vi "Image (Mask) SGL Data.vi"(8 "error in (no error)":errorcluster, 10 "Image Mask Refnum":T2, 11 "Src Image Refnum":T2) -> (0 "error out":errorcluster, 1 "% of Image":dbl, 2 "[Pixel Coordinates]":T1[](array[typedef]), 3 "Pixel Values(Float)":sgl[](array[numeric]), 4 "# Mask Pixels":i32, 5 "CPU (s)":dbl)   [LabVIEW 2021]
doc: "Returns the value (SGL) of pixels od the <B>Src Image</B> matching the mask.\n<B>Image Mask</B> needs to be of U8 or U16 type."
uses:
  <vilib>/vision/Image Controls.llb/IMAQ Image.ctl
  Image Point.ctl
  <vilib>/vision/NI_Vision_Development_Module.lvlib
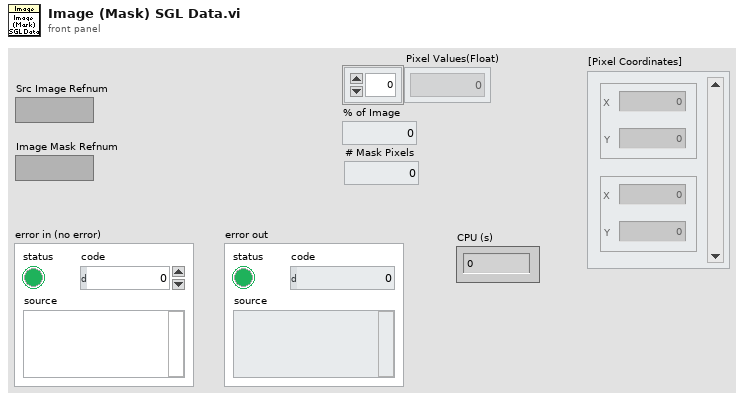
[diagram p1: front panel]
types:
  T1 = typedef "Image Point.ctl" = cluster{"X":i32, "Y":i32}
  T2 = typedef "IMAQ Image.ctl" = refnum<image>
  T3 = typedef "Image Type" = u32
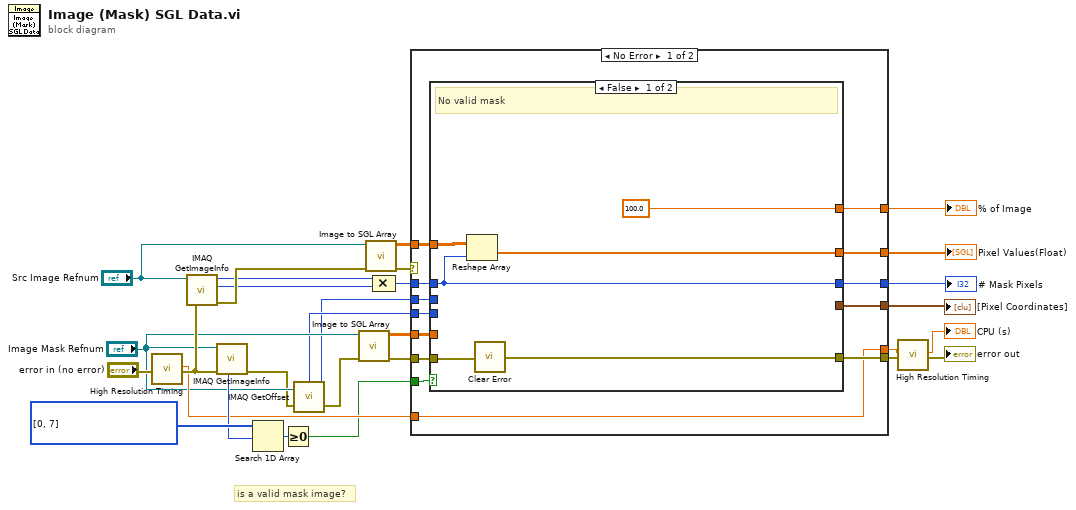
[diagram p0: block diagram]
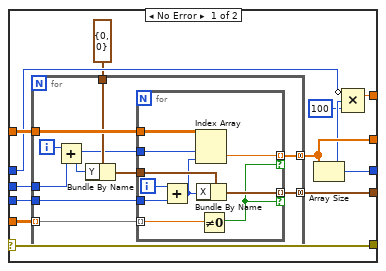
[diagram p3: hidden frame]
diagram:
  w29 = T3[] [0, 7] items=["Grayscale (U8)", "Grayscale (I16)", "Grayscale (SGL)", "Complex (CSG)", "RGB (U32)", "HSL (U32)", "RGB (U64)", "Grayscale (U16)"] ("Array")
  # "is a valid mask image?"
  n1 = call "High Resolution Timing.vi"("Error In"="error in (no error)") -> ("elapsed (relative) seconds"=w13:dbl, "Error Out"=w17:errorcluster)  [unwired: 16 in, 1 out]
  n2 = call "IMAQ GetImageInfo"("error in (no error)"=w17, "Image"="Src Image Refnum") -> ("error out"=w26:errorcluster, "Y Resolution"=w23:i32, "X Resolution"=w24:i32)  [unwired: 2 in, 5 out]
  n3 = call "IMAQ GetImageInfo"("error in (no error)"=w17, "Image"="Image Mask Refnum") -> ("error out"=w9:errorcluster, "Image Type"=w28:T3)  [unwired: 2 in, 6 out]
  n4 = Search 1D Array(1D array=w29, element=w28) -> (index of element=w27:i32)  [unwired: 1 in]
  n5 = Greater Or Equal To 0?(x=w27) -> (x >= 0?=w5:bool)
  n6 = call "IMAQ GetOffset"("Image"="Image Mask Refnum", "error in (no error)"=w9) -> ("Y Offset"=w7:i32, "X Offset"=w8:i32, "error out"=w6:errorcluster)  [unwired: 2 in]
  n7 = call "Image to SGL Array.vi"("error in (no error)"=w6, "Image"="Image Mask Refnum") -> ("error out"=w22:errorcluster, "Image Pixels (Float)"=w19:sgl[][])  [unwired: 8 in]
  n8 = call "Image to SGL Array.vi"("error in (no error)"=w26, "Image"="Src Image Refnum") -> ("error out"=w16:errorcluster, "Image Pixels (Float)"=w21:sgl[][])  [unwired: 8 in]
  n9 = Compound Arithmetic op=MULTIPLY(w24, w23) -> (w20:i32)
  n10 = case shown="No Error" w16 {
    selector: w16 -> [_ w95]
    tunnel: w5 -> [w42 _]
    tunnel: w22 -> [w41 _]
    tunnel: w21 -> [w38 _]
    tunnel: w20 -> [w40 _]
    tunnel: w19 -> [w39 _]
    tunnel: [w35 w95] -> w15
    tunnel: [w34 w94] -> w12
    tunnel: w13 -> [w34 w94]
    tunnel: w8 -> [w36 _]
    tunnel: w7 -> [w37 _]
    tunnel: [w33 _] -> w4
    tunnel: [w32 _] -> w3
    tunnel: [w31 _] -> w2
    tunnel: [w30 _] -> w1
    frame No Error {
      n11 = case shown="False" w42 {
        tunnel: w40 -> [w44 w57]
        tunnel: [w44 w56] -> w31
        tunnel: w41 -> [w47 w54]
        tunnel: [w43 w58] -> w33
        tunnel: w39 -> [_ w59]
        tunnel: [sgl 100.0 ("% of Image") w55] -> w32
        tunnel: [w46 w53] -> w35
        tunnel: w38 -> [w45 w52]
        tunnel: w37 -> [_ w51]
        tunnel: w36 -> [_ w50]
        tunnel: [_ w49] -> w30
        frame False {
          # "No valid mask"
          n12 = Reshape Array(w45, w44) -> (w43:sgl[])
          n13 = call "Clear Error.vi"("Error In"=w47) -> ("no Error Out"=w46:errorcluster)  [unwired: 8 in]
        }
        frame True {
          # "use mask"
          n14 = case shown="Error .." w54 {
            selector: w54 -> [w71 w93]
            tunnel: w59 -> [w70 _]
            tunnel: w52 -> [w69 _]
            tunnel: [w66 _] -> w58
            tunnel: w57 -> [w64 w92]
            tunnel: [w65 w92] -> w56
            tunnel: [w63 _] -> w55
            tunnel: [w71 w93] -> w53
            tunnel: w51 -> [w68 _]
            tunnel: w50 -> [w67 _]
            tunnel: [w60 _] -> w49
            frame No Error {
              n15 = for {
                tunnel: w70 -> [w81] mode=indexing
                tunnel: w69 -> [w80]
                tunnel: w68 -> [w78]
                tunnel: w67 -> [w77]
                tunnel: [w76] -> w66 mode=concatenating
                tunnel: T1 {"X"=0, "Y"=0} ("[Pixel Coordinates]") -> [w74]
                tunnel: [w72] -> w60 mode=concatenating
                i -> [w79]
                n16 = Add(x=w79, y=w78) -> (x+y=w73:i32)
                n17 = Bundle By Name(cluster=w74, "Y"=w73) -> (w75:T1)
                n18 = for {
                  tunnel: w81 -> [w87] mode=indexing
                  tunnel: w80 -> [w91]
                  tunnel: w73 -> [w90]
                  tunnel: w77 -> [w88]
                  tunnel: [w86] -> w76 mode=indexing if=w82
                  tunnel: w75 -> [w85]
                  tunnel: [w83] -> w72 mode=indexing if=w82
                  i -> [w89]
                  n19 = Add(x=w89, y=w88) -> (x+y=w84:i32)
                  n20 = Index Array(array=w91, index (row)=w90, index (col)=w84) -> (element=w86:sgl)
                  n21 = Bundle By Name(cluster=w85, "X"=w84) -> (w83:T1)
                  n22 = Not Equal To 0?(x=w87) -> (x != 0?=w82:bool)
                }
              }
              n23 = Array Size(array=w66) -> (size(s)=w65:i32)
              n24 = Compound Arithmetic op=MULTIPLY(invert w64, w65, 100 ("value")) -> (w63:dbl)
            }
            frame Error {
            }
          }
        }
      }
    }
    frame Error {
    }
  }
  "Pixel Values(Float)" <- w4
  "% of Image" <- w3
  "# Mask Pixels" <- w2
  "[Pixel Coordinates]" <- w1
  n25 = call "High Resolution Timing.vi"("relative seconds (NaN)"=w12, "Error In"=w15) -> ("elapsed (relative) seconds"=→"CPU (s)":dbl, "Error Out"=→"error out":errorcluster)  [unwired: 15 in, 1 out]
